vi "User Calibration New.vi"(9 "output cluster 3":T3 {"Current Settings"."Pump" items=["Pump 0", "Pump 1", "Pump 2", "Pump 3", "Pump 4", "Pump 5"]; "Current Settings"."Chart X axis Timescale" min=20 max=180 step=1; "Current Settings"."RunTime Mode Settings"."Exp. Gas Tank" items=["0.07", "0.031", "0.877", "1.863", "3.881", "5.790", "7.688", "6.000"]; "Current Settings"."RunTime Mode Settings"."Insp. Gas Tank" items=["0.07", "0.031", "0.877", "1.863", "3.881", "5.790", "7.688", "6.000"]; "Current Settings"."RunTime Mode Settings"."I:E Ratio" max=30 scale=0.0..7.0; "Current Settings"."RunTime Mode Settings"."Resp Rate Brpm" min=0 max=30 format="%.2f"; "Current Settings"."TE#2 Configuration"."Serial Port"."XOFF Char" format="%.0x"; "Current Settings"."TE#2 Configuration"."Serial Port"."XON Char" format="%.0x"; "Current Settings"."TE#2 Configuration"."Serial Port"."flow control" items=["None"=0, "XON/XOFF"=1, "RTS/CTS"=2, "DTR/DSR"=4]; "Current Settings"."TE#2 Configuration"."Serial Port"."stop bits" items=["1.0"=10, "1.5"=15, "2.0"=20]; "Current Settings"."TE#2 Configuration"."Serial Port"."data bits" min=5 max=8 step=1; "Current Settings"."TE#2 Configuration"."Serial Port"."baud rate" items=["75"=75, "110"=110, "134"=134, "150"=150, "300"=300, "600"=600, "1200"=1200, "1800"=1800, "2400"=2400, "4800"=4800, "7200"=7200, "9600"=9600, "14400"=14400, "19200"=19200, "28800"=28800, "38400"=38400, "56000"=56000, "57600"=57600, "115200"=115200, "128000"=128000, "230400"=230400]; "Current Settings"."TE#2 Configuration"."Serial Port"."termination char" format="%.0x"; "Current Settings"."TE#1 Configuration"."Serial Port"."XOFF Char" format="%.0x"; "Current Settings"."TE#1 Configuration"."Serial Port"."XON Char" format="%.0x"; "Current Settings"."TE#1 Configuration"."Serial Port"."flow control" items=["None"=0, "XON/XOFF"=1, "RTS/CTS"=2, "DTR/DSR"=4]; "Current Settings"."TE#1 Configuration"."Serial Port"."stop bits" items=["1.0"=10, "1.5"=15, "2.0"=20]; "Current Settings"."TE#1 Configuration"."Serial Port"."data bits" min=5 max=8 step=1; "Current Settings"."TE#1 Configuration"."Serial Port"."baud rate" items=["75"=75, "110"=110, "134"=134, "150"=150, "300"=300, "600"=600, "1200"=1200, "1800"=1800, "2400"=2400, "4800"=4800, "7200"=7200, "9600"=9600, "14400"=14400, "19200"=19200, "28800"=28800, "38400"=38400, "56000"=56000, "57600"=57600, "115200"=115200, "128000"=128000, "230400"=230400]; "Current Settings"."TE#1 Configuration"."Serial Port"."termination char" format="%.0x"; "Current Settings"."Capnometer Configuration"."Device" items=["None", "TidalWave", "LoFlow / Canary", "Capnogard"]; "Current Settings"."Capnometer Configuration"."Serial Port"."XOFF Char" format="%.0x"; "Current Settings"."Capnometer Configuration"."Serial Port"."XON Char" format="%.0x"; "Current Settings"."Capnometer Configuration"."Serial Port"."flow control" items=["None"=0, "XON/XOFF"=1, "RTS/CTS"=2, "DTR/DSR"=4]; "Current Settings"."Capnometer Configuration"."Serial Port"."stop bits" items=["1.0"=10, "1.5"=15, "2.0"=20]; "Current Settings"."Capnometer Configuration"."Serial Port"."data bits" min=5 max=8 step=1; "Current Settings"."Capnometer Configuration"."Serial Port"."baud rate" items=["75"=75, "110"=110, "134"=134, "150"=150, "300"=300, "600"=600, "1200"=1200, "1800"=1800, "2400"=2400, "4800"=4800, "7200"=7200, "9600"=9600, "14400"=14400, "19200"=19200, "28800"=28800, "38400"=38400, "56000"=56000, "57600"=57600, "115200"=115200, "128000"=128000, "230400"=230400]; "Current Settings"."Capnometer Configuration"."Serial Port"."termination char" format="%.0x"; "Current Settings"."DAQx Settings"."Analog Output Settings (Volts)" format="%#.3g"; "Current Settings"."DAQx Settings"."Duty Cycle" min=10.0 max=90.0 format="%.1g"; "Current Settings"."DAQx Settings"."Frequency" min=20.0 max=200.0; "Current Settings"."DataLogging Settings"."Data File Duration (Minutes)" min=2 max=200 format="%#.2g"; "Current Settings"."Calibration Settings"."Tolerance #2" min=2 max=4096; "Current Settings"."Calibration Settings"."Cal. Average" min=2 max=4096; "Current Settings"."Test Settings"."Test Sensor ID" items=["(select)", "RB", "YC", "", "Other"]}) -> (3 "Exit":bool)   [LabVIEW 2016]
uses:
  Controls/Pump Settings.ctl
  Controls/DAQ Needed.ctl
  Controls/Processed Variables.ctl
  Controls/AirPump Controls.ctl
  Controls/IE Ratio knob.ctl
  Controls/UI Settings.ctl
  Controls/Aux CO2 Control.ctl
  Controls/Serial Visa Control.ctl
  Controls/Aux CO2 Selector.ctl
  Controls/Aux TE Control.ctl
  Controls/Queues And Others.ctl
  Controls/Cal Refs.ctl
  Miscellaneous/Globals.vi
panel:
  out "stage 5 - offset adjust":i16[][](array[numeric])=[[0, 3, 500, 1, 1], [1, 3, 500, 1, 1], [2, 3, 500, 1, 1], [3, 3, 500, 1, 1], [4, 3, 500, 1, 1], [5, 3, 500, 1, 1], [6, 3, 500, 1, 1], [7, 3, 500, 0, 0], [8, 3, 500, 0, 0], [9, 3, 500, 0, 0], [10, 3, 500, 0, 0], [11, 3, 500, 0, 0], [12, 3, 500, 0, 0], [13, 3, 500, 0, 0], [14, 3, 500, 0, 0], [15, 3, 500, 0, 0], [16, 3, 500, 0, 0], [17, 3, 500, 0, 0], [18, 3, 500, 0, 0], [19, 3, 500, 0, 0], [20, 3, 500, 0, 0], [21, 3, 500, 0, 0], [22, 3, 500, 0, 0], [23, 3, 500, 0, 0], [24, 3, 500, 0, 0], [25, 3, 500, 0, 0], [26, 3, 500, 0, 0], [27, 3, 500, 0, 0], [28, 3, 500, 0, 0], [29, 3, 500, 0, 0], [30, 3, 500, 0, 0], [31, 3, 500, 0, 0], [32, 3, 500, 0, 0], [33, 3, 500, 0, 0], [34, 3, 500, 0, 0], [35, 3, 500, 0, 0], [36, 3, 500, 0, 0], [37, 3, 500, 0, 0], [38, 3, 500, 0, 0], [39, 3, 500, 0, 0], [40, 3, 500, 0, 0], [41, 3, 500, 0, 0], [42, 3, 500, 0, 0], [43, 3, 500, 0, 0], [44, 3, 500, 0, 0], [45, 3, 500, 0, 0], [46, 3, 500, 0, 0], [47, 3, 500, 0, 0], [48, 3, 500, 0, 0], [49, 3, 500, 0, 0], [50, 3, 500, 0, 0], [51, 3, 500, 0, 0], [52, 3, 500, 0, 0], [53, 3, 500, 0, 0], [54, 3, 500, 0, 0], [55, 3, 500, 0, 0], [56, 3, 500, 0, 0], [57, 3, 500, 0, 0], [58, 3, 500, 0, 0], [59, 3, 500, 0, 0], [60, 3, 500, 0, 0], [61, 3, 500, 0, 0], [62, 3, 500, 0, 0], [63, 3, 500, 0, 0], [64, 3, 500, 0, 0], [65, 3, 500, 0, 0], [66, 3, 500, 0, 0], [67, 3, 500, 0, 0], [68, 3, 500, 0, 0], [69, 3, 500, 0, 0], [70, 3, 500, 0, 0], [71, 3, 500, 0, 0], [72, 3, 500, 0, 0], [73, 3, 500, 0, 0], [74, 3, 500, 0, 0], [75, 3, 500, 0, 0], [76, 3, 500, 0, 0], [77, 3, 500, 0, 0], [78, 3, 500, 0, 0], [79, 3, 500, 0, 0], [80, 3, 500, 0, 0], [81, 3, 500, 0, 0], [82, 3, 500, 0, 0], [83, 3, 500, 0, 0], [84, 3, 500, 0, 0], [85, 3, 500, 0, 0], [86, 3, 500, 0, 0], [87, 3, 500, 0, 0], [88, 3, 500, 0, 0], [89, 3, 500, 0, 0], [90, 3, 500, 0, 0], [91, 3, 500, 0, 0], [92, 3, 50, 1, 1]]
  in  "Humidity Status 2":refnum<vi>
  in  "output cluster":T1
  out "Cluster":T2={"Tcal_Chamber"=0.0, "Tcal_PCB"=nan, "Tcal_Film"=0.0, "Tcal_Humidity"=0.0, "Tcal_Det"=[], "Cal Gas"=nan, "Reference"=0.0} {"Reference" format="%.3g"; "Cal Gas" format="%.3g"; "Tcal_Det" format="%.2f"; "Tcal_Humidity" format="%.2f"; "Tcal_Film" format="%.2f"; "Tcal_PCB" format="%.2f"; "Tcal_Chamber" format="%.2f"}
  out "Pump Settings":T11
  out "Error":bool
  out "Index":u16
  out "null array":i16[][](array[numeric])
  out "stage 4 - span":i16[][](array[numeric])=[[0, 3, 500, 1, 1], [1, 3, 500, 1, 1], [2, 3, 500, 1, 1], [3, 3, 500, 1, 1], [4, 3, 500, 1, 1], [5, 3, 500, 1, 1], [6, 3, 500, 1, 1], [7, 3, 500, 0, 0], [8, 3, 500, 0, 0], [9, 3, 500, 0, 0], [10, 3, 500, 0, 0], [11, 3, 500, 0, 0], [12, 3, 500, 0, 0], [13, 3, 500, 0, 0], [14, 3, 500, 0, 0], [15, 3, 500, 0, 0], [16, 3, 500, 0, 0], [17, 3, 500, 0, 0], [18, 3, 500, 0, 0], [19, 3, 500, 0, 0], [20, 3, 500, 0, 0], [21, 3, 500, 0, 0], [22, 3, 500, 0, 0], [23, 3, 500, 0, 0], [24, 3, 500, 0, 0], [25, 3, 500, 0, 0], [26, 3, 500, 0, 0], [27, 3, 500, 0, 0], [28, 3, 500, 0, 0], [29, 3, 500, 0, 0], [30, 3, 500, 0, 0], [31, 3, 500, 0, 0], [32, 3, 500, 0, 0], [33, 3, 500, 0, 0], [34, 3, 500, 0, 0], [35, 3, 500, 0, 0], [36, 3, 500, 0, 0], [37, 3, 500, 0, 0], [38, 3, 500, 0, 0], [39, 3, 500, 0, 0], [40, 3, 500, 0, 0], [41, 3, 500, 0, 0], [42, 3, 500, 0, 0], [43, 3, 500, 0, 0], [44, 3, 500, 0, 0], [45, 3, 500, 0, 0], [46, 3, 500, 0, 0], [47, 3, 500, 0, 0], [48, 3, 500, 0, 0], [49, 3, 500, 0, 0], [50, 3, 500, 0, 0], [51, 3, 500, 0, 0], [52, 3, 500, 0, 0], [53, 3, 500, 0, 0], [54, 3, 500, 0, 0], [55, 3, 500, 0, 0], [56, 3, 500, 0, 0], [57, 3, 500, 0, 0], [58, 3, 500, 0, 0], [59, 3, 500, 0, 0], [60, 3, 500, 0, 0], [61, 3, 500, 0, 0], [62, 3, 500, 0, 0], [63, 3, 500, 0, 0], [64, 3, 500, 0, 0], [65, 3, 500, 0, 0], [66, 3, 500, 0, 0], [67, 3, 500, 0, 0], [68, 3, 500, 0, 0], [69, 3, 500, 0, 0], [70, 3, 500, 0, 0], [71, 3, 500, 0, 0], [72, 3, 500, 0, 0], [73, 3, 500, 0, 0], [74, 3, 500, 0, 0], [75, 3, 500, 0, 0], [76, 3, 500, 0, 0], [77, 3, 500, 0, 0], [78, 3, 500, 0, 0], [79, 3, 500, 0, 0], [80, 3, 500, 0, 0], [81, 3, 500, 0, 0], [82, 3, 500, 0, 0], [83, 3, 500, 0, 0], [84, 3, 500, 0, 0], [85, 3, 500, 0, 0], [86, 3, 500, 0, 0], [87, 3, 500, 0, 0], [88, 3, 500, 0, 0], [89, 3, 500, 0, 0], [90, 3, 500, 0, 0], [91, 3, 500, 0, 0], [92, 3, 50, 1, 1]]
  out "stage 3 - high":i16[][](array[numeric])=[[0, 3, 500, 0, 1], [1, 3, 500, 0, 1], [2, 3, 500, 0, 1], [3, 3, 500, 0, 1], [4, 3, 500, 0, 1], [5, 3, 500, 0, 1], [6, 3, 50, 0, 1]]
  out "stage 2 - zeroing":i16[][](array[numeric])=[[0, 2, 500, 1, 0], [1, 2, 500, 1, 0], [2, 2, 500, 1, 0], [3, 2, 500, 1, 0], [4, 2, 500, 1, 0], [5, 2, 500, 1, 0], [6, 2, 50, 1, 0]]
  out "stage1 - humidity check":i16[][](array[numeric])=[[0, 1, 500, 1, 0], [1, 1, 50, 1, 0], [2, 1, 50, 1, 0], [3, 1, 50, 1, 0], [4, 1, 50, 1, 0], [5, 1, 50, 1, 0], [6, 1, 100, 0, 1], [7, 1, 150, 0, 1], [8, 1, 200, 0, 1], [9, 1, 250, 1, 0], [10, 1, 300, 1, 1], [0, 1, 350, 0, 0]]
  out "DAC Currents":sgl[](array[numeric]) caption="Currents" format="%.4g"
  out "Raw_Humidity":dbl format="%.2f"
  out "Raw Chamber":dbl format="%.2f"
  in  "Quit":bool
  out "Calibration Complete":bool
  out "Progress":u16(slide) scale=0.0..666.0
  out "CalStatusTab":T12(tab)
  in  "Skip Cal":bool
  in  "OK  7":bool
  in  "Calgas":dbl caption="Calibration Gas Concentration" format="%.2g"
  out "start time":timestamp format="%<%H:%M:%S>T"
  in  "Gas Tank":u8=5
  out "Calibration Message":enum16{"Calibration Is Required - "}(ring)
  in  "Calibration Code":T13(ring)
  out "Stable":bool
  in  "Low Humidity Threshold (%)":u16=60
  in  "Hi Humidity Threshold (%)":u16=90
  in  "Humidity Status":T14(ring)
  out "Stablizing":dbl[][](graph)
  out "Cal Fail":bool
  out "Cluster 2":T15 {"D'" format="%0.4f"; "C'" format="%0.4f"; "B'" format="%0.4f"; "A'" format="%0.4f"; "D" format="%0.4f"; "C" format="%0.4f"; "B" format="%0.4f"; "A" format="%0.4f"; "V_span(target)" format="%0.4f"; "V_6d(target)" format="%0.4f"; "V_0d(target)" format="%0.4f"; "C6FC2V" format="%0.4f"; "C0FC2V" format="%0.4f"}
  out "Cluster 3":T16 {"DAC scale" format="%.3g"; "mI" format="%.3g"; "V_RA(15mA)" format="%0.4f"; "V_RA(5mA)" format="%0.4f"}
  out "Zero":dbl[][](graph)
  out "Zero Status":T17(ring)
  out "delta 2":dbl=nan caption="delta" format="%.3g"
  out "Cluster 4":T18 {"mI 2" format="%.3g"; "V_RA(15mA) 2" format="%0.4f"; "V_RA(5mA) 2" format="%0.4f"}
  out "Zero 3":dbl[][](graph)
  out "delta 3":dbl=nan caption="delta" format="%.3g"
  out "Zero Status 2":T19(ring)
  in  "OK 9":bool
  out "DAC":u16[](array[numeric]) format="%03x"
  out "V_Span Delta":dbl[](array[numeric]) format="%0.4f"
  out "Span Good":bool[](array[boolean])
  out "I'mBlue":bool[](array[boolean]) caption="BlueLED"
  out "Span Point Calibration":dbl[][](graph)
  out "delta":dbl=nan format="%.3g"
  out "Zero Offset":dbl[][](graph)
  in  "OK 10":bool
  out "Calibration Complete -":timestamp format="%<%H:%M:%S\n%m/%d/%y>T"
  out "duration":i16 caption="mins" format="%<%H:%M:%S>t"
  out "Cluster 5":T20 {"Gain(adjust)" format="%0.4f"; "V_span(adjust)" format="%0.4f"; "V_0(adjust)\ncal offsets" format="%0.4f"; "V_span(ImA)" format="%0.4f"; "V_6d(ImA)\nActual" format="%0.4f"; "V_0d(ImA)\nActual" format="%0.4f"}
  out "CalGasTank":u8=5 max=7
  out "elapsed time":i16 format="%<%H:%M:%S>t"
  # "Channel 1"
  # "Channel 2"
  # "Channel 3"
  # "Channel 4"
  # "Note: Setting Brpm to zero will\ndisable Insp / Exp digital output."
  # "mmHg"
  # "pts"
  # "tolerance"
  # "AN5 (Temp 1)"
  # "AN6 (Temp 2)"
  # "AN7 (Temp 3)"
  # "AN8 (T FET)"
  # "AN0 (T POT)"
  # "Tref (Set Pt))"
  # "(Spare)"
  # "Initializing"
  # "1. Please Place Freespira On Base-Station\n \n2. Attach Cannula and Breathe Normally \n \n3. Enter Calibration Gas Concentration \n \n4. Press OK To Begin Calibration Process"
  # "Please Enter Calibration Code"
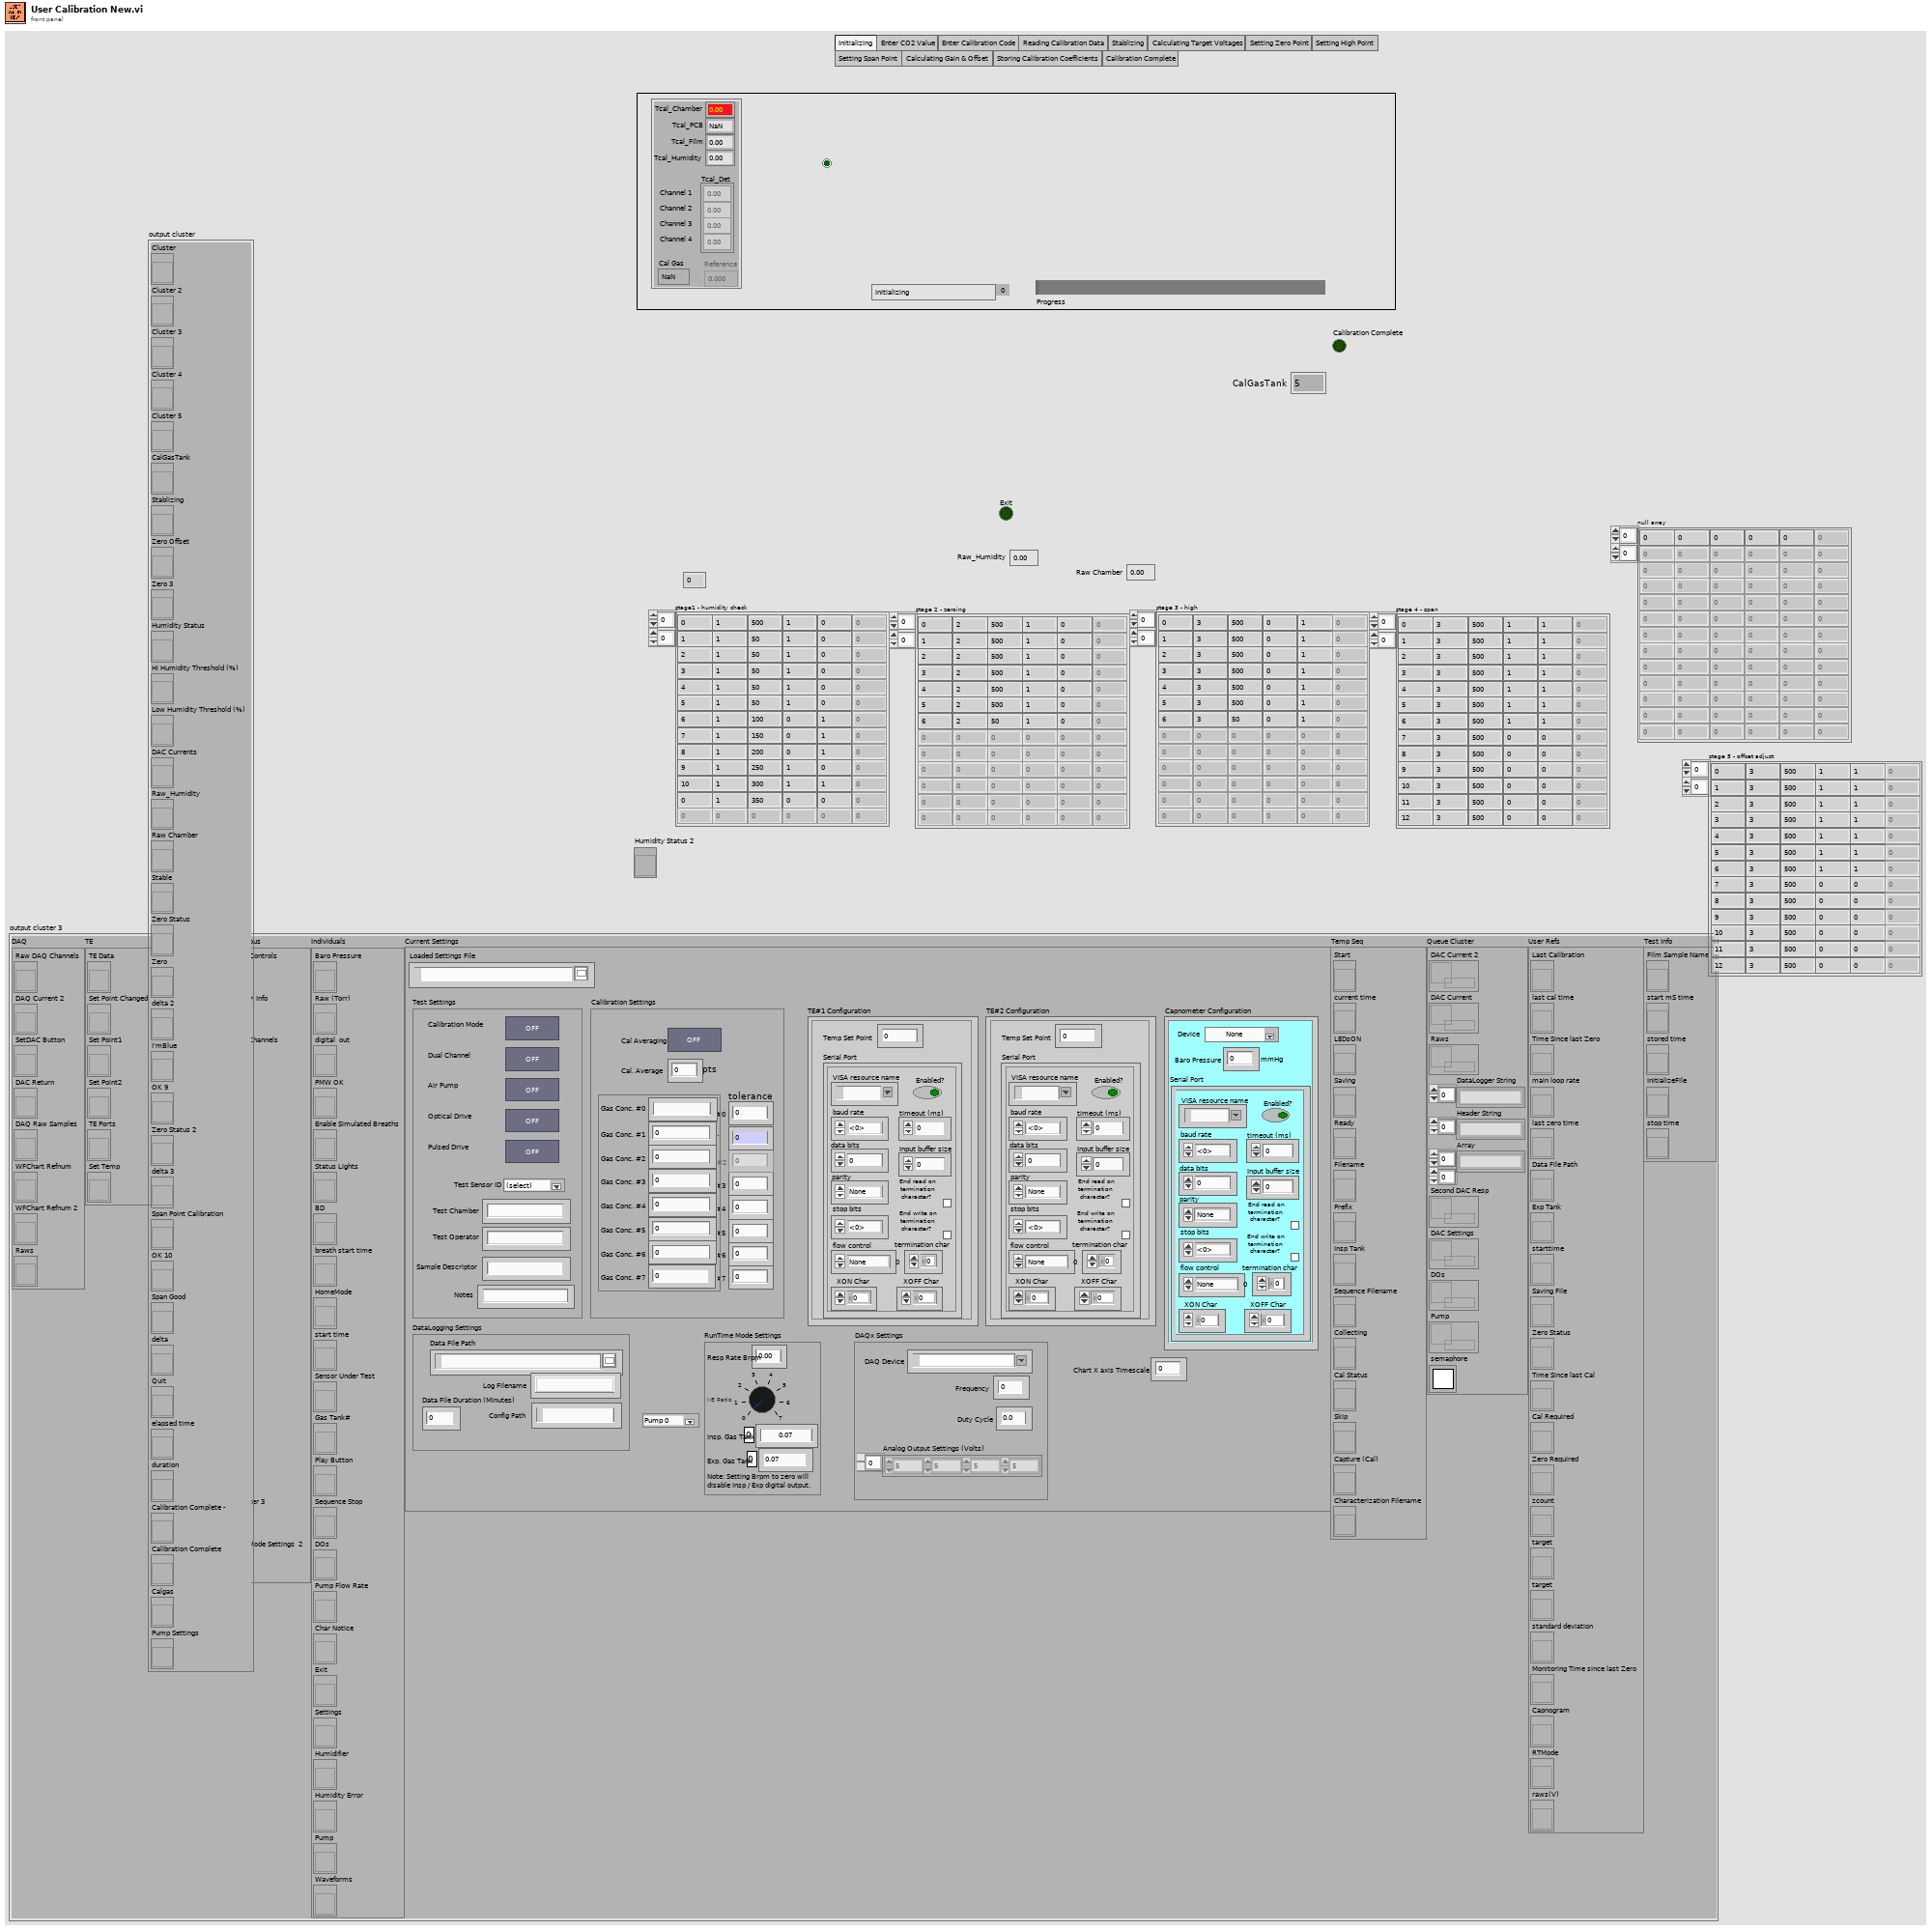
[diagram p1: front panel]
types:
  T1 = typedef "Cal Refs.ctl" = cluster{"Cluster":refnum<vi>, "Cluster 2":refnum<vi>, "Cluster 3":refnum<vi>, "Cluster 4":refnum<vi>, "Cluster 5":refnum<vi>, "CalGasTank":refnum<vi>, "Stablizing":refnum<vi>, "Zero Offset":refnum<vi>, "Zero 3":refnum<vi>, "Humidity Status":refnum<vi>, "Hi Humidity Threshold (%)":refnum<vi>, "Low Humidity Threshold (%)":refnum<vi>, "DAC Currents":refnum<vi>, "Raw_Humidity":refnum<vi>, "Raw Chamber":refnum<vi>, "Stable":refnum<vi>, "Zero Status":refnum<vi>, "Zero":refnum<vi>, "delta 2":refnum<vi>, "I'mBlue":refnum<vi>, "OK 9":refnum<vi>, "Zero Status 2":refnum<vi>, "delta 3":refnum<vi>, "Span Point Calibration":refnum<vi>, "OK 10":refnum<vi>, "Span Good":refnum<vi>, "delta":refnum<vi>, "Quit":refnum<vi>, "elapsed time":refnum<vi>, "duration":refnum<vi>, "Calibration Complete -":refnum<vi>, "Calibration Complete":refnum<vi>, "Calgas":refnum<vi>, "Pump Settings":refnum<vi>}
  T2 = cluster{"Tcal_Chamber":dbl, "Tcal_PCB":dbl, "Tcal_Film":dbl, "Tcal_Humidity":dbl, "Tcal_Det":dbl[], "Cal Gas":dbl, "Reference":dbl}
  T3 = typedef "DAQ Needed.ctl" = cluster{"DAQ":cluster{"Raw DAQ Channels":refnum<vi>, "DAQ Current 2":refnum<vi>, "SetDAC Button":refnum<vi>, "DAC Return":refnum<vi>, "DAQ Raw Samples":refnum<vi>, "WFChart Refnum":refnum<vi>, "WFChart Refnum 2":refnum<vi>, "Raws":refnum<vi>}, "TE":cluster{"TE Data":refnum<vi>, "Set Point Changed":refnum<vi>, "Set Point1":refnum<vi>, "Set Point2":refnum<vi>, "TE Ports":refnum<vi>, "Set Temp":refnum<vi>}, "Loflo":cluster{"Loflo":refnum<vi>, "Saving Data":refnum<vi>, "Zero":refnum<vi>, "Zero 2":refnum<vi>, "Ready to Log 2":refnum<vi>, " sequence":refnum<vi>, "Loflo Status ":refnum<vi>, "Aux CO2 Port":refnum<vi>}, "Miscellaneous":cluster{"Air Pump Controls":refnum<vi>, "Application Info":refnum<vi>, "Detector Channels ":refnum<vi>, "Cluster":refnum<vi>, "Cluster2":refnum<vi>, "Cluster3":refnum<vi>, "Cluster4":refnum<vi>, "Cluster 5":refnum<vi>, "Cluster 6":refnum<vi>, "Cluster 7":refnum<vi>, "Logging":refnum<vi>, "Cluster 10":refnum<vi>, "Cluster 8":refnum<vi>, "DAQ Cluster 3":refnum<vi>, "RunTime Mode Settings  2":refnum<vi>}, "Individuals":cluster{"Baro Pressure":refnum<vi>, "Raw (Torr)":refnum<vi>, "digital  out":refnum<vi>, "PMW OK":refnum<vi>, "Enable Simulated Breaths":refnum<vi>, "Status Lights":refnum<vi>, "BD":refnum<vi>, "breath start time":refnum<vi>, "HomeMode":refnum<vi>, "start time":refnum<vi>, "Sensor Under Test":refnum<vi>, "Gas Tank#":refnum<vi>, "Play Button":refnum<vi>, "Sequence Stop":refnum<vi>, "DOs":refnum<vi>, "Pump Flow Rate":refnum<vi>, "Char Notice":refnum<vi>, "Exit":refnum<vi>, "Settings":refnum<vi>, "Humidifier":refnum<vi>, "Humidity Error":refnum<vi>, "Pump":refnum<vi>, "Waveforms":refnum<vi>}, "Current Settings":T4, "Temp Seq":cluster{"Start":refnum<vi>, "current time":refnum<vi>, "LEDsON":refnum<vi>, "Saving":refnum<vi>, "Ready":refnum<vi>, "Filename":refnum<vi>, "Prefix":refnum<vi>, "Insp Tank":refnum<vi>, "Sequence Filename":refnum<vi>, "Collecting":refnum<vi>, "Cal Status":refnum<vi>, "Skip":refnum<vi>, "Capture (Cal)":refnum<vi>, "Characterization Filename":refnum<vi>}, "Queue Cluster":T9, "User Refs":cluster{"Last Calibration":refnum<vi>, "last cal time":refnum<vi>, "Time Since last Zero":refnum<vi>, "main loop rate":refnum<vi>, "last zero time":refnum<vi>, "Data File Path":refnum<vi>, "Exp Tank":refnum<vi>, "starttime":refnum<vi>, "Saving File":refnum<vi>, "Zero Status":refnum<vi>, "Time Since last Cal":refnum<vi>, "Cal Required":refnum<vi>, "Zero Required":refnum<vi>, "zcount":refnum<vi>, "target":refnum<vi>, "target":refnum<vi>, "standard deviation":refnum<vi>, "Monitoring Time since last Zero":refnum<vi>, "Capnogram":refnum<vi>, "RTMode":refnum<vi>, "raws(V)":refnum<vi>}, "Test Info":cluster{"Film Sample Name":refnum<vi>, "start mS time":refnum<vi>, "stored time":refnum<vi>, "InitializeFile":refnum<vi>, "stop time":refnum<vi>}}
  T4 = typedef "UI Settings.ctl" = cluster{"Loaded Settings File":path, "Test Settings":cluster{"Dual Channel":bool, "Air Pump":bool, "Optical Drive":bool, "Pulsed Drive":bool, "Calibration Mode":bool, "Test Sensor ID":u16, "Test Chamber":string, "Test Operator":string, "Sample Descriptor":string, "Notes":string}, "Calibration Settings":cluster{"Cal. Average":u16, "Cal Averaging":bool, "Tolerance #0":sgl, "Tolerance #7":sgl, "Tolerance #6":sgl, "Tolerance #5":sgl, "Tolerance #4":sgl, "Tolerance #3":sgl, "Tolerance #2":sgl, "Tolerance #1":sgl, "Gas Tank Settings":cluster{"Gas Conc. #0":string, "Gas Conc. #1":sgl, "Gas Conc. #2":sgl, "Gas Conc. #3":sgl, "Gas Conc. #4":sgl, "Gas Conc. #5":sgl, "Gas Conc. #6":sgl, "Gas Conc. #7":sgl}}, "DataLogging Settings":cluster{"Data File Path":path, "Data File Duration (Minutes)":sgl, "Log Filename":string, "Config Path":path}, "DAQx Settings":cluster{"DAQ Device":tag, "Frequency":dbl, "Duty Cycle":dbl, "Analog Output Settings (Volts)":sgl[]}, "Capnometer Configuration":T5, "TE#1 Configuration":T8, "TE#2 Configuration":T8, "RunTime Mode Settings ":cluster{"Resp Rate Brpm ":sgl, "I:E Ratio":u8, "Insp. Gas Tank":u16, "Exp. Gas Tank":u16}, "Chart X axis Timescale":u16, "Pump":u16}
  T5 = typedef "Aux CO2 Control.ctl" = cluster{"Serial Port":T6, "Baro Pressure":u32, "Device":T7}
  T6 = typedef "Serial Visa Control.ctl" = cluster{"termination char":u8, "End read on termination character?":bool, "Enabled?":bool, "VISA resource name":refnum<visa-resource-name>, "baud rate":u32, "data bits":u16, "parity":enum16{"None", "Odd", "Even", "Mark", "Space"}, "stop bits":u16, "flow control":u16, "timeout (ms)":u32, "Input buffer size":u32, "End write on termination character?":bool, "XON Char":u8, "XOFF Char":u8}
  T7 = typedef "Aux CO2 Selector.ctl" = u16
  T8 = typedef "Aux TE Control.ctl" = cluster{"Temp Set Point":sgl, "Serial Port":T6}
  T9 = typedef "Queues And Others.ctl" = cluster{"DAC Current 2":refnum<queue>, "DAC Current":refnum<queue>, "Raws":refnum<queue>, "DataLogger String":string[], "Header String":string[], "Array":string[][], "Second DAC Resp":refnum<queue>, "DAC Settings":refnum<queue>, "DOs":refnum<queue>, "Pump":refnum<queue>, "semaphore":T10}
  T10 = typedef "Semaphore RefNum" = refnum<k1>
  T11 = typedef "Pump Settings.ctl" = cluster{"Flow":u16, "Solenoid#1":bool, "Solenoid#2":bool, "ignore":bool}
  T12 = enum32{"Initializing", "Enter CO2 Value", "Enter Calibration Code", "Reading Calibration Data", "Stablizing", "Calculating Target Voltages", "Setting Zero Point", "Setting High Point", "Setting Span Point", "Calculating Gain & Offset", "Storing Calibration Coefficients", "Calibration Complete"}
  T13 = enum8{"", "<User Defined>", "11111 - default", "22222 - MM_1_NS", "33333 - MM_2_S"}
  T14 = enum16{"Waiting For Film to Stabilize", "Film Stable", "Exiting", "Initializing"}
  T15 = cluster{"CalFile Selected":path, "TYPE":string, "DATE":string, "C0FC2V":dbl[], "C6FC2V":dbl[], "V_0d(target)":dbl[], "V_6d(target)":dbl[], "V_span(target)":dbl[], "CHANNEL":string[], "Status":bool[], "BlueLED 2":bool[], "C2V":u8[], "A":dbl[], "B":dbl[], "C":dbl[], "D":dbl[], "V2C":u8[], "A'":dbl[], "B'":dbl[], "C'":dbl[], "D'":dbl[]}
  T16 = cluster{"CHANNEL 2":string[], "BlueLED":bool[], "V_RA(5mA)":dbl[], "V_RA(15mA)":dbl[], "mI":dbl[], "DAC scale":dbl[]}
  T17 = enum16{"Setting Zero at 5 mA", "Setting Zero at 15 mA", "Calculating slopes"}
  T18 = cluster{"CHANNEL 3":string[], "BlueLED 3":bool[], "V_RA(5mA) 2":dbl[], "V_RA(15mA) 2":dbl[], "mI 2":dbl[]}
  T19 = enum16{"Setting High at 5 mA", "Setting High at 15 mA", "Calculating slopes"}
  T20 = cluster{"V_0d(ImA)\nActual":dbl[], "V_6d(ImA)\nActual":dbl[], "V_span(ImA)":dbl[], "V_0(adjust)\ncal offsets":dbl[], "V_span(adjust)":dbl[], "Gain(adjust)":dbl[]}
  T21 = enum32{"Invalid", "Standard", "Closed", "Hidden", "Minimized", "Maximized"}
  T22 = typedef "Processed Variables.ctl" = cluster{"Detector Chl 1":sgl, "Humidity":dbl, "Film Temperature":dbl, "Detector Chl 2":sgl, "Ref CO2":sgl, "Detector Chl 3":sgl, "Detector Chl 4":sgl, "Det. Temperature":dbl, "Bath Temperature":dbl, "Ambient Temperature":dbl, "rt Baro Pressure":u16, "Chamber Temperature":dbl}
  T23 = cluster{"Avg Hum":dbl, "Humidity":dbl, "Chamber Temperature":dbl, "Ref CO2":sgl, "Array":sgl[], "RawCO2s":dbl[], "ETCO2 Out":dbl, "RR Out":dbl, "BD":i32, bool}
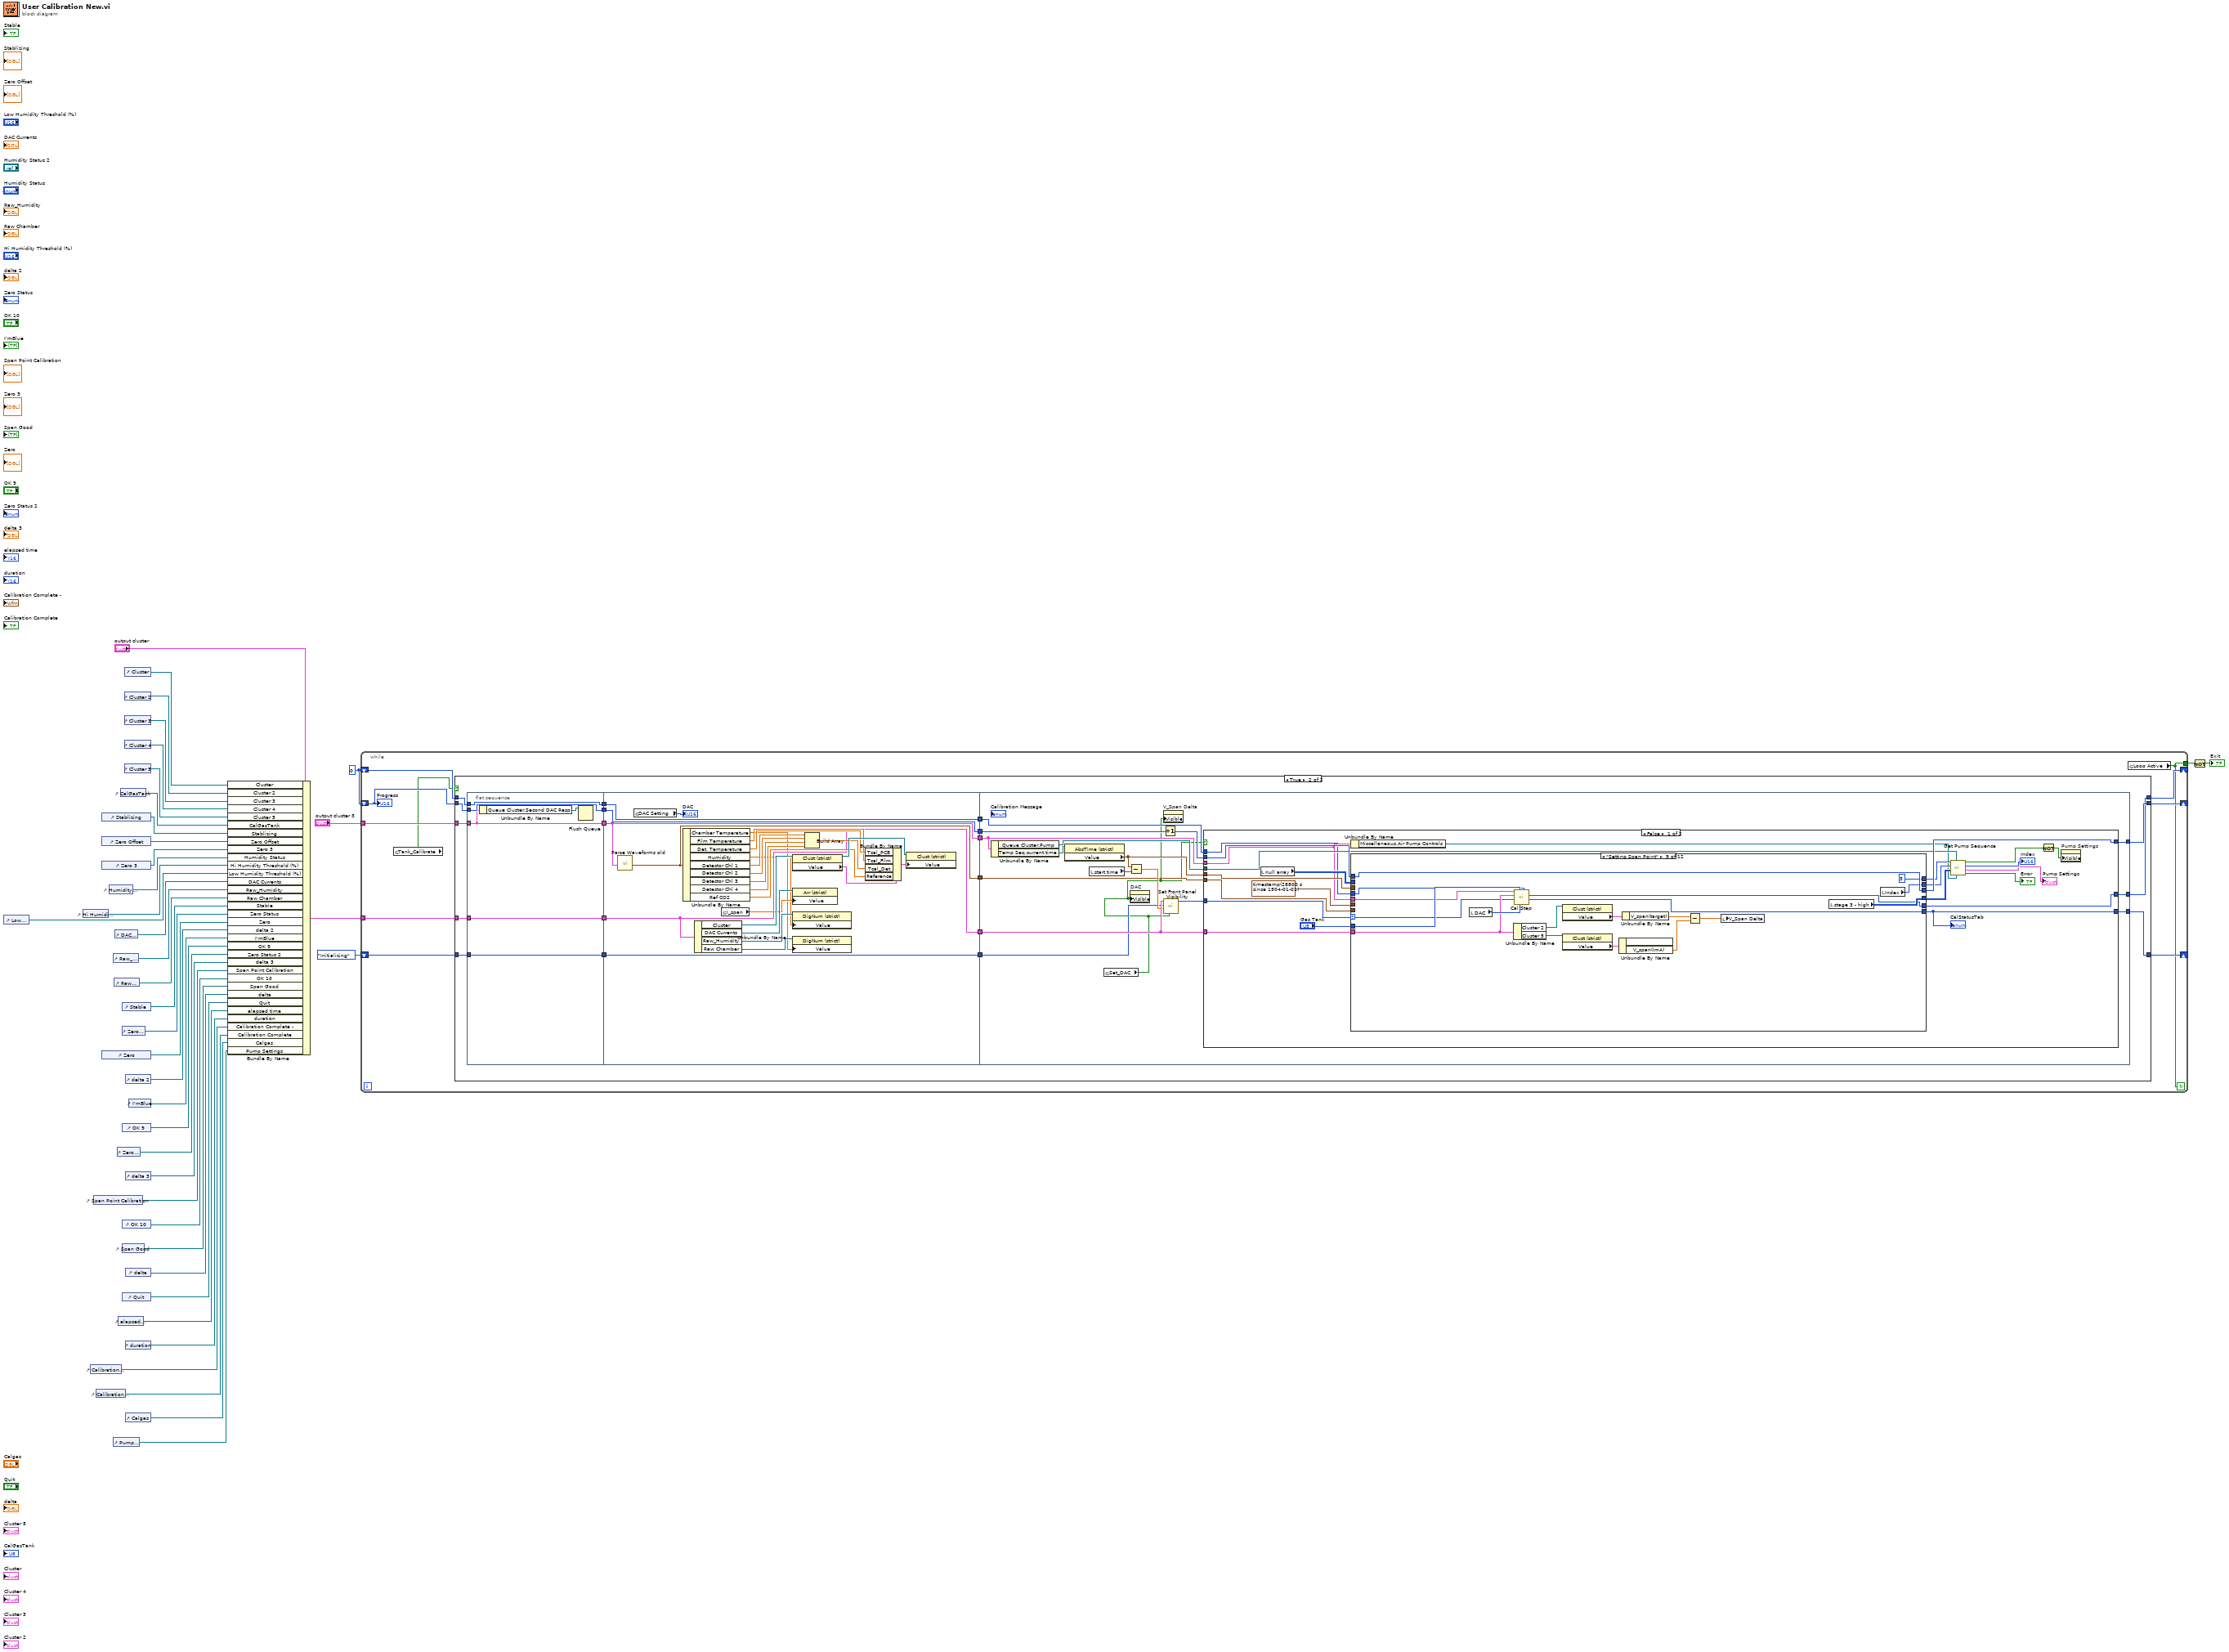
[diagram p0: block diagram]
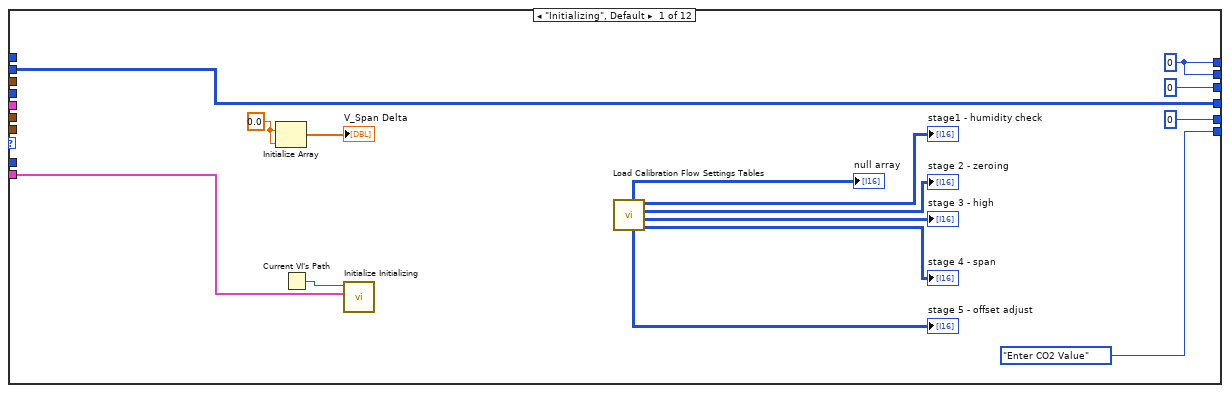
[diagram p3: hidden frame]
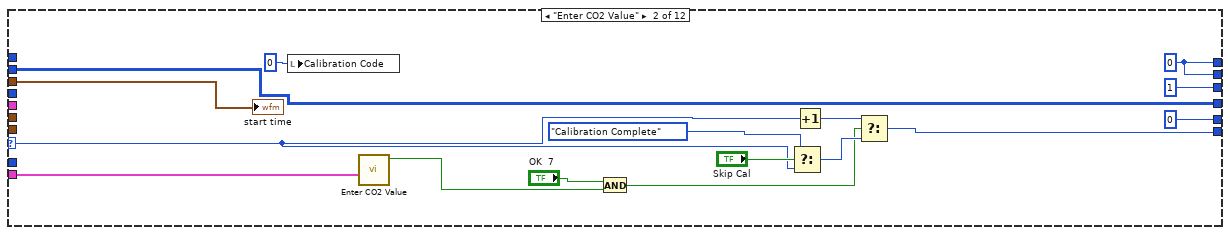
[diagram p4: hidden frame]
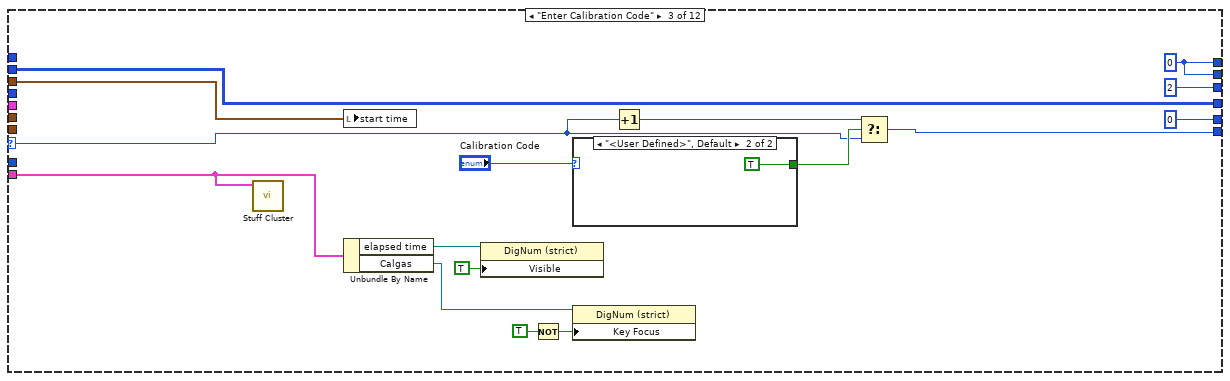
[diagram p5: hidden frame]
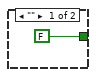
[diagram p6: hidden frame]
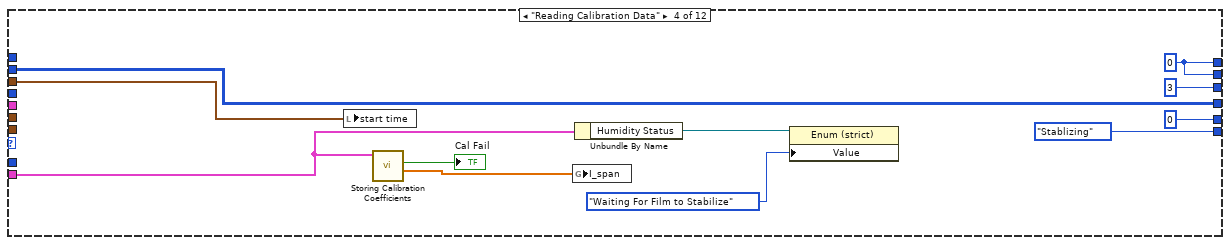
[diagram p7: hidden frame]
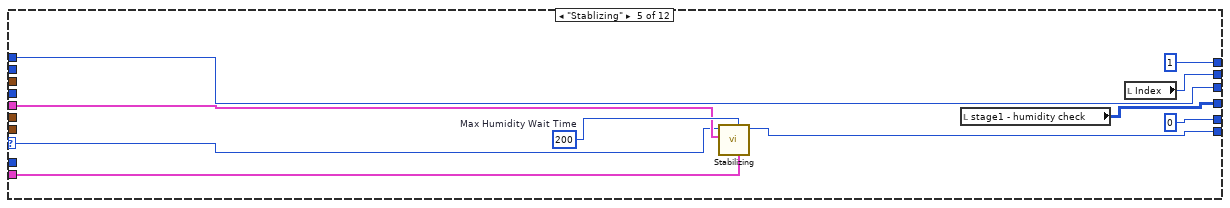
[diagram p8: hidden frame]
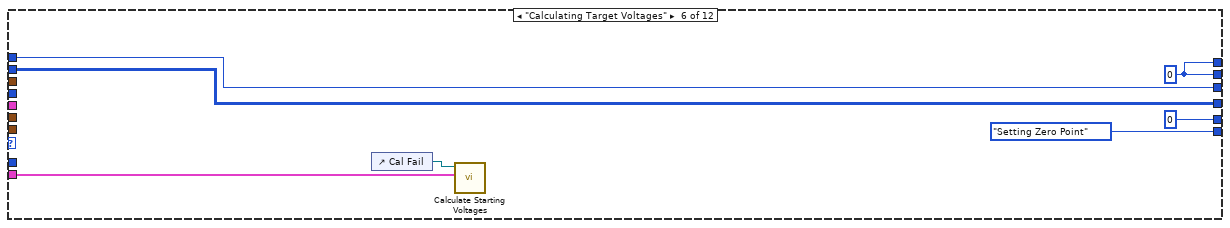
[diagram p9: hidden frame]
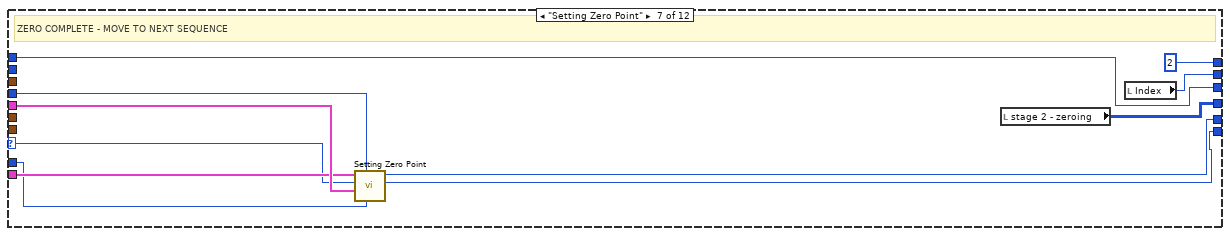
[diagram p10: hidden frame]
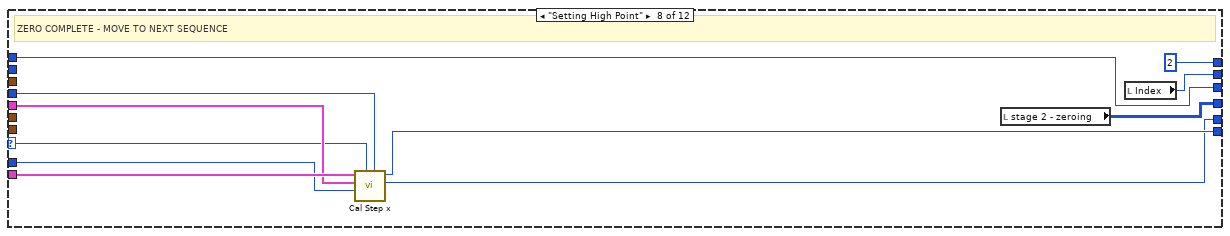
[diagram p11: hidden frame]
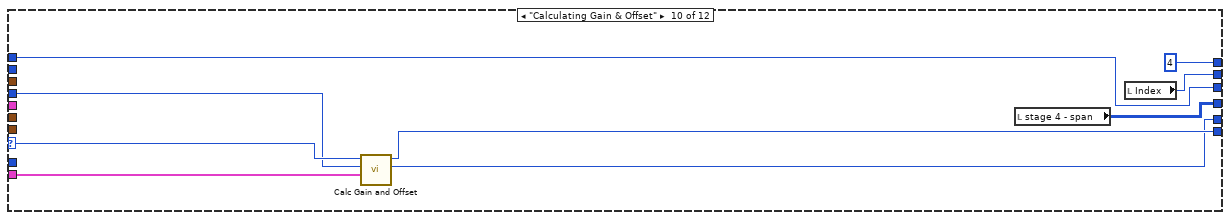
[diagram p12: hidden frame]
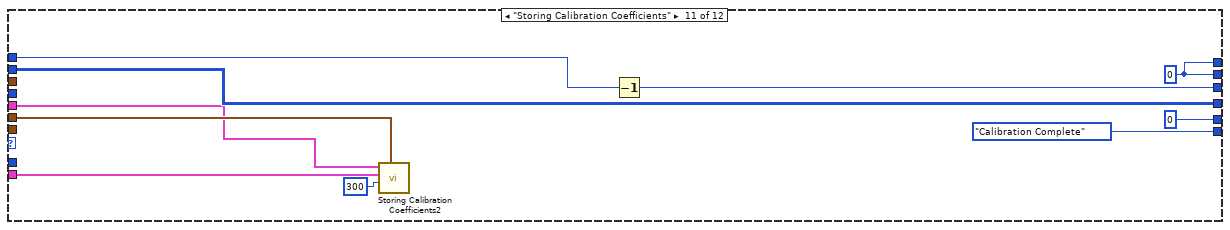
[diagram p13: hidden frame]
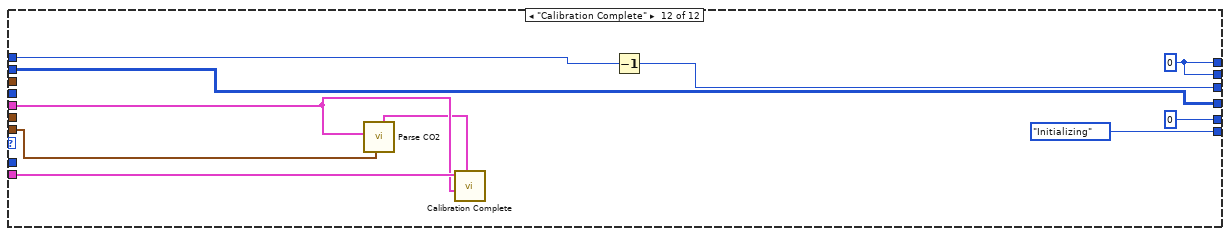
[diagram p14: hidden frame]
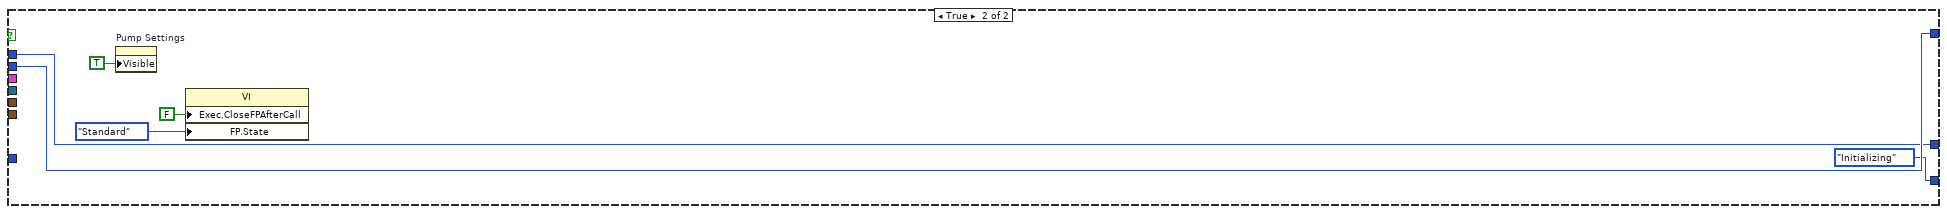
[diagram p15: hidden frame]
diagram:
  w3 = 0
  n1 = control-ref of="Low Humidity Threshold (%)"() -> (w27:refnum<vi>)
  n2 = control-ref of="Hi Humidity Threshold (%)"() -> (w28:refnum<vi>)
  n3 = control-ref of="Calibration Complete -"() -> (w8:refnum<vi>)
  n4 = control-ref of="Span Point Calibration"() -> (w15:refnum<vi>)
  n5 = control-ref of="Calibration Complete"() -> (w7:refnum<vi>)
  n6 = control-ref of="Stablizing"() -> (w32:refnum<vi>)
  n7 = control-ref of="Zero Offset"() -> (w31:refnum<vi>)
  n8 = control-ref of="Zero 3"() -> (w30:refnum<vi>)
  n9 = control-ref of="Zero"() -> (w21:refnum<vi>)
  n10 = control-ref of="Humidity Status"() -> (w29:refnum<vi>)
  n11 = control-ref of="Raw_Humidity"() -> (w25:refnum<vi>)
  n12 = control-ref of="Pump Settings"() -> (w5:refnum<vi>)
  n13 = control-ref of="Raw Chamber"() -> (w24:refnum<vi>)
  n14 = control-ref of="DAC Currents"() -> (w26:refnum<vi>)
  n15 = control-ref of="Zero Status 2"() -> (w17:refnum<vi>)
  n16 = control-ref of="elapsed time"() -> (w10:refnum<vi>)
  n17 = control-ref of="CalGasTank"() -> (w33:refnum<vi>)
  n18 = control-ref of="Stable"() -> (w23:refnum<vi>)
  n19 = control-ref of="Zero Status"() -> (w22:refnum<vi>)
  n20 = control-ref of="OK 9"() -> (w18:refnum<vi>)
  n21 = control-ref of="OK 10"() -> (w14:refnum<vi>)
  n22 = control-ref of="Span Good"() -> (w13:refnum<vi>)
  n23 = control-ref of="Quit"() -> (w11:refnum<vi>)
  n24 = control-ref of="Cluster"() -> (w41:refnum<vi>)
  n25 = control-ref of="Cluster 2"() -> (w40:refnum<vi>)
  n26 = control-ref of="Cluster 3"() -> (w39:refnum<vi>)
  n27 = control-ref of="Cluster 4"() -> (w38:refnum<vi>)
  n28 = control-ref of="Cluster 5"() -> (w34:refnum<vi>)
  n29 = control-ref of="delta 2"() -> (w20:refnum<vi>)
  n30 = control-ref of="delta 3"() -> (w16:refnum<vi>)
  n31 = control-ref of="delta"() -> (w12:refnum<vi>)
  n32 = control-ref of="duration"() -> (w9:refnum<vi>)
  n33 = control-ref of="Calgas"() -> (w6:refnum<vi>)
  n34 = control-ref of="I'mBlue"() -> (w19:refnum<vi>)
  n35 = Bundle By Name(cluster="output cluster", "Cluster"=w41, "Cluster 2"=w40, "Cluster 3"=w39, "Cluster 4"=w38, "Cluster 5"=w34, "CalGasTank"=w33, "Stablizing"=w32, "Zero Offset"=w31, "Zero 3"=w30, "Humidity Status"=w29, "Hi Humidity Threshold (%)"=w28, "Low Humidity Threshold (%)"=w27, "DAC Currents"=w26, "Raw_Humidity"=w25, "Raw Chamber"=w24, "Stable"=w23, "Zero Status"=w22, "Zero"=w21, "delta 2"=w20, "I'mBlue"=w19, "OK 9"=w18, "Zero Status 2"=w17, "delta 3"=w16, "Span Point Calibration"=w15, "OK 10"=w14, "Span Good"=w13, "delta"=w12, "Quit"=w11, "elapsed time"=w10, "duration"=w9, "Calibration Complete -"=w8, "Calibration Complete"=w7, "Calgas"=w6, "Pump Settings"=w5) -> (w36:T1)
  n36 = while {
    tunnel: w36 -> [w51]
    tunnel: "output cluster 3" -> [w50]
    shift-right: [w47] -> _
    shift-left: w3 -> [w48]
    shift-right: [w46] -> _
    shift-left: T12."Initializing" ("CalStatusTab") -> [w49]
    shift-right: [w44] -> _
    shift-left: w3 -> [w45]
    tunnel: [w43] -> w2
    stop <- w43 continue-if-true
    n37 = global read "Globals.vi" "Tank_Calibrate"() -> (w42:bool)
    n38 = case shown="True" w42 {
      tunnel: w48 -> [w53 w70]
      tunnel: w51 -> [_ w69]
      tunnel: w50 -> [_ w68]
      tunnel: [w54 w67] -> w46
      tunnel: w49 -> [w54 w64]
      tunnel: [w53 w66] -> w47
      tunnel: w45 -> [w52 w57]
      tunnel: [w52 w55] -> w44
      frame False {
      }
      frame True {
        n39 = flat-sequence {
          tunnel: w64 -> [w77]
          tunnel: w68 -> [w75]
          tunnel: w69 -> [w78]
          tunnel: w70 -> [w79]
          tunnel: [w79] -> w63
          tunnel: [w78] -> w62
          tunnel: [w75] -> w61
          tunnel: [w77] -> w60
          tunnel: [w74] -> w58
          tunnel: w57 -> [w74]
          tunnel: [w84] -> w73
          tunnel: [w92] -> w72
          tunnel: [w82] -> w71
          tunnel: [w83] -> w65
          tunnel: w63 -> [w84]
          tunnel: w62 -> [w92]
          tunnel: w61 -> [w82]
          tunnel: w60 -> [w83]
          tunnel: [w81] -> w59
          tunnel: w58 -> [w80]
          tunnel: [w80] -> w56
          tunnel: w73 -> [w118]
          tunnel: w72 -> [w117]
          tunnel: w71 -> [w109]
          tunnel: [w112] -> w67
          tunnel: [w111] -> w66
          tunnel: w65 -> [w110]
          tunnel: w59 -> [w108]
          tunnel: w56 -> [w107]
          tunnel: [w106] -> w55
          frame #0 {
            n40 = Unbundle By Name(w75) -> ("Queue Cluster.Second DAC Resp"=w76:refnum<queue>)
            n41 = Flush Queue(queue=w76) -> ()  [unwired: 1 in, 3 out]
          }
          frame #1 {
            n42 = call "Parse Waveforms old.vi"("Daq Needed"=w82) -> ("Processed Variables"=w81:T22)  [unwired: 5 in, 5 out]
            n43 = global read "Globals.vi" "DAC Setting"() -> (→"DAC":u16[])
            n44 = Unbundle By Name(w81) -> ("Chamber Temperature"=w85:dbl, "Film Temperature"=w95:dbl, "Det. Temperature"=w96:dbl, "Humidity"=w87:dbl, "Detector Chl 1"=w103:sgl, "Detector Chl 2"=w102:sgl, "Detector Chl 3"=w101:sgl, "Detector Chl 4"=w104:sgl, "Ref CO2"=w93:sgl)
            n45 = Unbundle By Name(w92) -> ("Cluster"=w91:refnum<vi>, "DAC Currents"=w90:refnum<vi>, "Raw_Humidity"=w88:refnum<vi>, "Raw Chamber"=w86:refnum<vi>)
            n46 = global read "Globals.vi" "I_span"() -> (w89:dbl[])
            n47 = property class="Clust (strict)"(reference=w91) -> (reference out=w99:refnum<vi>, "Value"=w98:T2)  [unwired: 1 in, 1 out]
            n48 = property class="Arr (strict)"(reference=w90, "Value"=w89) -> ()  [unwired: 1 in, 2 out]
            n49 = property class="DigNum (strict)"(reference=w88, "Value"=w87) -> ()  [unwired: 1 in, 2 out]
            n50 = property class="DigNum (strict)"(reference=w86, "Value"=w85) -> ()  [unwired: 1 in, 2 out]
            n51 = Build Array(w103, w102, w101, w104) -> (w94:sgl[])
            n52 = Bundle By Name(cluster=w98, "Tcal_PCB"=w96, "Tcal_Film"=w95, "Tcal_Det"=w94, "Reference"=w93) -> (w97:T2)
            n53 = property class="Clust (strict)"(reference=w99, "Value"=w97) -> ()  [unwired: 1 in, 2 out]
          }
          frame #2 {
            n54 = Unbundle By Name(w109) -> ("Queue Cluster.Pump"=w115:refnum<queue>, "Temp Seq.current time"=w114:refnum<vi>)
            n55 = property class="AbsTime (strict)"(reference=w114) -> ("Value"=w113:timestamp)  [unwired: 1 in, 2 out]
            n56 = local read "start time"() -> (w121:timestamp)
            n57 = global read "Globals.vi" "Set_DAC"() -> (w105:bool)
            n58 = Subtract(x=w113, y=w121) -> (x-y=w116:dbl)
            n59 = property on="DAC" class="Arr (strict)"("Visible"=w105) -> ()  [unwired: 2 in, 2 out]
            n60 = Increment(x=w118) -> (x+1=w119:i32)
            n61 = property on="V_Span Delta" class="Arr (strict)"("Visible"=w105) -> ()  [unwired: 2 in, 2 out]
            n62 = call "Set Front Panel Visibility.vi"("Set Value"=w105, "Elapsed Time"=w116, "Current Tab"=w110, "output cluster"=w117) -> ("New Tab"=w120:T12)  [unwired: 7 in]
            n63 = case shown="False" w105 {
              tunnel: [w144 w297] -> w111
              tunnel: w120 -> [w126 _]
              tunnel: w119 -> [w142 w297]
              tunnel: w113 -> [w131 _]
              tunnel: w117 -> [w132 _]
              tunnel: w109 -> [w129 _]
              tunnel: w115 -> [w130 _]
              tunnel: [w127 T12."Initializing" ("New Tab")] -> w112
              tunnel: w108 -> [w125 _]
              tunnel: w107 -> [w124 w292]
              tunnel: [w123 w292] -> w106
              frame False {
                n64 = local read "null array"() -> (w141:i16[][])
                n65 = Unbundle By Name(w129) -> ("Miscellaneous.Air Pump Controls"=w128:refnum<vi>)
                n66 = case shown="\"Setting Span Point\"" w126 {
                  selector: w126 -> [_ w161 w183 _ w207 _ w225 w236 w246 w266 _ _]
                  tunnel: w142 -> [_ _ _ _ w214 w221 w232 w243 w262 w271 w273 w291]
                  tunnel: [0 1 2 3 w214 w221 w232 w243 w262 w271 w272 w288] -> w144
                  tunnel: timestamp(28800 s since 1904-01-01) -> [_ _ _ _ _ _ _ _ _ _ w281 _]
                  tunnel: [w154 w173 w190 w203 w213 w220 w231 w242 w259 w270 w280 w290] -> w137
                  tunnel: w141 -> [w154 w173 w190 w203 _ w220 _ _ _ _ w280 w290]
                  tunnel: [w153 w170 w189 w202 1 w219 2 ("Count") 2 ("Count") 3 ("Count") 4 ("Count") w279 w289] -> w140
                  tunnel: [w153 w170 w189 w202 w212 w219 w229 w240 w258 w269 w279 w289] -> w139
                  tunnel: w131 -> [_ w172 w188 w201 _ _ _ _ _ _ _ _]
                  tunnel: "Gas Tank" -> [_ _ _ _ _ _ w226 w237 w256 _ _ _]
                  tunnel: w132 -> [w152 w171 w176 w195 w210 w218 w227 w239 w252 w267 w277 w287]
                  tunnel: w129 -> [_ _ _ _ w208 _ w228 w238 w248 _ w278 w284]
                  tunnel: [T12."Enter CO2 Value" ("NewCalStatus") w162 w182 T12."Stablizing" ("Value") w206 T12."Setting Zero Point" ("NewCalStatus") w224 w235 w247 w265 T12."Calibration Complete" ("NewCalStatus") T12."Initializing" ("NewCalStatus")] -> w127
                  tunnel: w125 -> [_ _ _ _ _ _ _ _ _ _ _ w285]
                  tunnel: w124 -> [_ _ _ _ _ _ w223 w234 w245 w263 _ _]
                  tunnel: [u8 0 ("Count out") u8 0 ("Count out") u16 0 ("New Count") u8 0 ("New Count") u16 0 ("New Count") u16 0 ("New Count") w222 w233 w244 w264 u16 0 ("New Count") u16 0 ("New Count")] -> w123
                  frame "Initializing", Default {
                    w150 = 0.0
                    w153 = 0
                    n67 = Initialize Array(w150, w150) -> (→"V_Span Delta":dbl[])
                    n68 = Current VI's Path() -> (path=w145:path)
                    n69 = call "Initialize Initializing.vi"("output cluster"=w152, "path"=w145) -> ()  [unwired: 10 in]
                    n70 = call "Load Calibration Flow Settings Tables.vi"() -> ("stage 4 - span"=→"stage 4 - span":i16[][], "stage 3 - high"=→"stage 3 - high":i16[][], "stage 2 - zeroing"=→"stage 2 - zeroing":i16[][], "stage1 - humidity check"=→"stage1 - humidity check":i16[][], "stage 5 - offset adjust"=→"stage 5 - offset adjust":i16[][], "termination array - should be just one row of zeros"=→"null array":i16[][])  [unwired: 6 in]
                  }
                  frame "Enter CO2 Value" {
                    w170 = u8 0
                    n71 = local write "Calibration Code"(0) -> ()
                    n72 = call "Enter CO2 Value.vi"("output cluster"=w171) -> ("Good CO2"=w164:bool)  [unwired: 10 in]
                    n73 = And(x="OK  7", y=w164) -> (x .and. y?=w168:bool)
                    n74 = Select(t=T12."Calibration Complete" ("Value"), s="Skip Cal", f=w161) -> (s? t:f=w169:T12)
                    n75 = Increment(x=w161) -> (x+1=w167:T12)
                    n76 = Select(t=w167, s=w168, f=w169) -> (s? t:f=w162:T12)
                    "start time" <- w172
                  }
                  frame "Enter Calibration Code" {
                    w189 = u8 0
                    n77 = call "Stuff Cluster.vi"("output cluster"=w176) -> ()  [unwired: 10 in, 1 out]
                    n78 = local write "start time"(w188) -> ()
                    n79 = Unbundle By Name(w176) -> ("elapsed time"=w180:refnum<vi>, "Calgas"=w181:refnum<vi>)
                    n80 = property on="Property Node" class="DigNum (strict)"(reference=w180, "Visible"=TRUE) -> ()  [unwired: 1 in, 2 out]
                    n81 = Not(x=TRUE ("Key Focus")) -> (.not. x?=w178:bool)
                    n82 = case shown="\"<User Defined>\", Default" "Calibration Code" {
                      tunnel: [FALSE TRUE] -> w186
                      frame "" {
                      }
                      frame "<User Defined>", Default {
                      }
                    }
                    n83 = property on="Property Node" class="DigNum (strict)"(reference=w181, "Key Focus"=w178) -> ()  [unwired: 1 in, 2 out]
                    n84 = Increment(x=w183) -> (x+1=w185:T12)
                    n85 = Select(t=w185, s=w186, f=w183) -> (s? t:f=w182:T12)
                  }
                  frame "Reading Calibration Data" {
                    w202 = u8 0
                    n86 = local write "start time"(w201) -> ()
                    n87 = call "Storing Calibration Coefficients.vi"("output cluster"=w195) -> ("Array"=w196:dbl[], "Error"=→"Cal Fail":bool)  [unwired: 9 in]
                    n88 = global write "Globals.vi" "I_span"(w196) -> ()
                    n89 = Unbundle By Name(w195) -> ("Humidity Status"=w198:refnum<vi>)
                    n90 = property class="Enum (strict)"(reference=w198, "Value"=enum16{"Waiting For Film to Stabilize"}."Waiting For Film to Stabilize" ("Enum")) -> ()  [unwired: 1 in, 2 out]
                  }
                  frame "Stablizing" {
                    w209 = 200  # Max Humidity Wait Time
                    n91 = call "Stabilizing.vi"("output cluster"=w210, "Max Humidity Wait Time"=w209, "output cluster 3"=w208, "CalStatus"=w207) -> ("NewCalStatus"=w206:T12)  [unwired: 7 in]
                    n92 = local read "stage1 - humidity check"() -> (w213:i16[][])
                    n93 = local read "Index"() -> (w212:u16)
                  }
                  frame "Calculating Target Voltages" {
                    w219 = u8 0 ("Count")
                    n94 = control-ref of="Cal Fail"() -> (w217:refnum<vi>)
                    n95 = call "Calculate Starting Voltages.vi"("output cluster"=w218, "Boolean in"=w217) -> ()  [unwired: 10 in]
                  }
                  frame "Setting Zero Point" {
                    # "ZERO COMPLETE - MOVE TO NEXT SEQUENCE"
                    n96 = call "Setting Zero Point.vi"("Gas Tank"=w226, "Count"=w223, "output cluster 3"=w228, "CalStatus"=w225, "output cluster"=w227) -> ("NewCalStatus"=w224:T12, "Count out"=w222:u8)  [unwired: 5 in]
                    n97 = local read "stage 2 - zeroing"() -> (w231:i16[][])
                    n98 = local read "Index"() -> (w229:u16)
                  }
                  frame "Setting High Point" {
                    # "ZERO COMPLETE - MOVE TO NEXT SEQUENCE"
                    n99 = call "Cal Step x.vi"("Count"=w234, "CalStatus"=w236, "Gas Tank"=w237, "output cluster 3"=w238, "output cluster"=w239) -> ("New Count"=w233:u8, "NewCalStatus"=w235:T12)  [unwired: 5 in]
                    n100 = local read "stage 2 - zeroing"() -> (w242:i16[][])
                    n101 = local read "Index"() -> (w240:u16)
                  }
                  frame "Setting Span Point" {
                    n102 = local read "DAC"() -> (w260:u16[])
                    n103 = Unbundle By Name(w252) -> ("Cluster 2"=w250:refnum<vi>, "Cluster 5"=w253:refnum<vi>)
                    n104 = call "Cal Step.vi"("Count"=w245, "DAC"=w260, "Gas Tank"=w256, "CalStatus"=w246, "output cluster"=w252, "output cluster 3"=w248) -> ("NewCalStatus"=w247:T12, "New Count"=w244:u8)  [unwired: 4 in]
                    n105 = property class="Clust (strict)"(reference=w250) -> ("Value"=w251:T15)  [unwired: 1 in, 2 out]
                    n106 = property class="Clust (strict)"(reference=w253) -> ("Value"=w255:T20)  [unwired: 1 in, 2 out]
                    n107 = Unbundle By Name(w255) -> ("V_span(ImA)"=w254:dbl[])  [unwired: 1 out]
                    n108 = Unbundle By Name(w251) -> ("V_span(target)"=w249:dbl[])
                    n109 = Subtract(x=w249, y=w254) -> (x-y=w261:dbl[])
                    n110 = local write "V_Span Delta"(w261) -> ()
                    n111 = local read "stage 3 - high"() -> (w259:i16[][])
                    n112 = local read "Index"() -> (w258:u16)
                  }
                  frame "Calculating Gain & Offset" {
                    n113 = call "Calc Gain and Offset.vi"("output cluster"=w267, "Count"=w263, "CalStatus"=w266) -> ("New Count"=w264:u8, "NewCalStatus"=w265:T12)  [unwired: 7 in]
                    n114 = local read "stage 4 - span"() -> (w270:i16[][])
                    n115 = local read "Index"() -> (w269:u16)
                  }
                  frame "Storing Calibration Coefficients" {
                    w279 = 0
                    n116 = call "Storing Calibration Coefficients2.vi"("Time Stamp"=w281, "Lo Flow in"=u16 300, "output cluster"=w277, "output cluster 3"=w278) -> ()  [unwired: 8 in]
                    n117 = Decrement(x=w273) -> (x-1=w272:i32)
                  }
                  frame "Calibration Complete" {
                    w289 = 0 ("Count")
                    n118 = call "Parse CO2.vi"("Processed Variables"=w285, "Daq Needed"=w284) -> ("output cluster"=w283:T23)  [unwired: 8 in, 1 out]
                    n119 = call "Calibration Complete.vi"("output cluster 2"=w283, "output cluster 3"=w284, "output cluster"=w287) -> ()  [unwired: 9 in]
                    n120 = Decrement(x=w291) -> (x-1=w288:i32)
                  }
                }
                "CalStatusTab" <- w127
                n121 = call "Get Pump Sequence.vi"("Miscellaneous.Air Pump Controls"=w128, "queue"=w130, "Array"=w137, "Index"=w139, "Stage"=w140) -> ("Error"=→"Error":bool, "Pump Settings"=→"Pump Settings":T11, "Updated Index"=→"Index":u16, "Ignore"=w134:bool)  [unwired: 3 in]
                n122 = Not(x=w134) -> (.not. x?=w133:bool)
                n123 = property on="Pump Settings" class="Clust (strict)"("Visible"=w133) -> ()  [unwired: 2 in, 2 out]
              }
              frame True {
                n124 = property on="Pump Settings" class="Clust (strict)"("Visible"=TRUE) -> ()  [unwired: 2 in, 2 out]
                n125 = property class="VI"("Exec.CloseFPAfterCall"=FALSE ("Calibration Complete"), "FP.State"=T21."Standard" ("Front Panel Window:State")) -> ()  [unwired: 2 in, 2 out]
              }
            }
          }
        }
      }
    }
    n126 = global read "Globals.vi" "Loop Active"() -> (w43:bool)
    "Progress" <- w48
  }
  n127 = Not(x=w2) -> (.not. x?=→"Exit":bool)
